vi "ThetaConversion.vi"(10 "Input rad":dbl format="%#_13g") -> (0 "out new":dbl)   [LabVIEW 2025]
panel:
  out "Waveform Chart":dbl(graph)
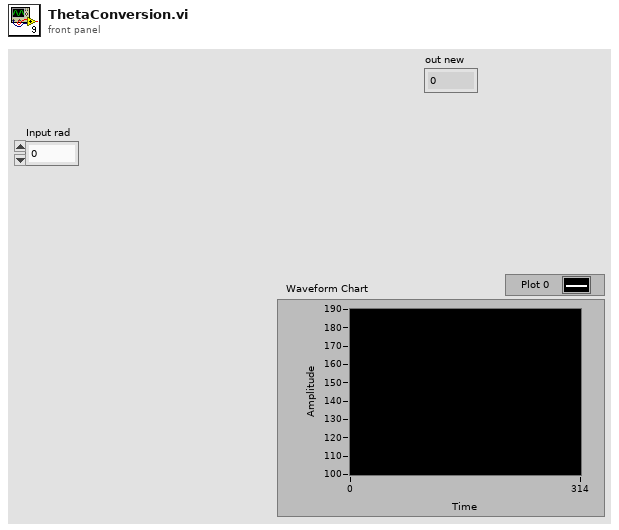
[diagram p1: front panel]
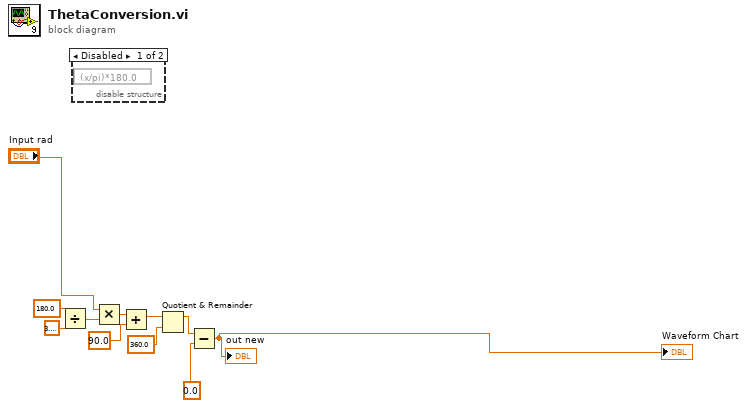
[diagram p0: block diagram]
diagram:
  n1 = Divide(x=180.0, y=3.141592653589793) -> (x/y=w9:dbl)
  n2 = disable-structure shown="Disabled" {
    frame Disabled {
      n3 = expression code="(x/pi)*180.0" ("radians to degrees")() -> ()  [unwired: 1 in, 1 out]
    }
    frame Enabled {
    }
  }
  n4 = Multiply(x="Input rad", y=w9) -> (x*y=w7:dbl)
  n5 = Add(x=w7, y=90.0) -> (x+y=w5:dbl)
  n6 = Quotient & Remainder(x=w5, y=360.0) -> (x-y*floor(x/y)=w2:dbl)  [unwired: 1 out]
  n7 = Subtract(x=w2, y=0.0) -> (x-y=→"Waveform Chart" →"out new":dbl)
